vi "ADXL345.vi"() -> ()   [LabVIEW 2012]
uses:
  <vilib>/LabVIEW Interface for Arduino/Type Defs/Board Type.ctl
  <vilib>/LabVIEW Interface for Arduino/LabVIEW Interface for Arduino.lvlib
panel:
  out "Scaled Accelerometer Data":dynamicdata(graph)
  out "Z-Tilt":dbl
  out "Y-Tilt":dbl
  out "X-Tilt":dbl
  out "Raw Accelerometer Data":T1
  in  "Z- Axis Gain":dbl
  in  "Y-Axis Gain":dbl
  in  "X-Axis Gain":dbl
  in  "Board Type (Uno)":T2=enum."Mega 2560"
  in  "Baud Rate (115200)":u32=57600
  in  "COM Port":refnum<visa-resource-name>
  in  "stop":bool
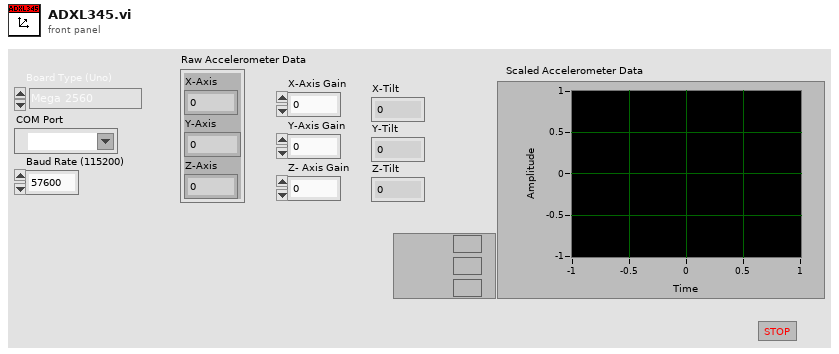
[diagram p1: front panel]
types:
  T1 = cluster{"X-Axis":i32, "Y-Axis":i32, "Z-Axis":i32}
  T2 = typedef "LabVIEW Interface for Arduino.lvlib/Board Type.ctl" = enum16{"Uno", "Dimuelanove w/Atmega 328", "Mega 2560"}
  T3 = typedef "LabVIEW Interface for Arduino.lvlib/Arduino Resource.ctl" = cluster{"VISA resource":refnum<visa-resource-name>, "Board Type":T2, "Connection Type":enum8{"USB / Serial"}, "Bytes Per Packet (15)":u8}
  T4 = cluster{"X-Tilt":dbl, "Y-Tilt":dbl, "Z-Tilt":dbl}
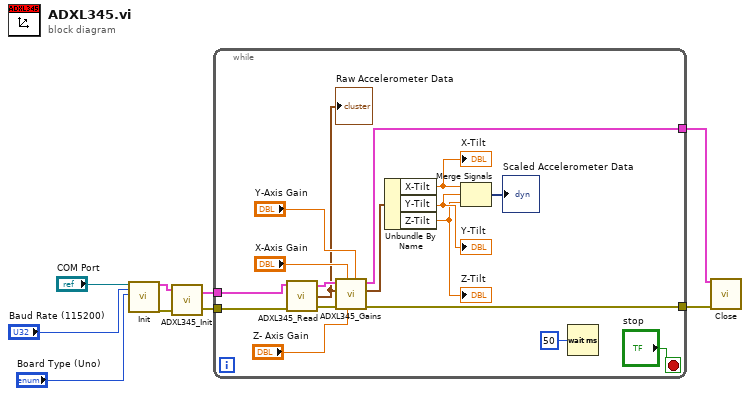
[diagram p0: block diagram]
diagram:
  n1 = call <vilib>:"Init.vi"("VISA resource"="COM Port", "Baud Rate (115200)"="Baud Rate (115200)", "Board Type (Uno)"="Board Type (Uno)") -> ("Arduino Resource"=w6:T3, "error out"=w5:errorcluster)  [unwired: 15 in]
  n2 = call "ADXL345_Init.vi"("error in"=w5, "Arduino Resource"=w6) -> ("error out"=w3:errorcluster, "Arduino Resource"=w4:T3)  [unwired: 1 in]
  n3 = while {
    tunnel: w4 -> [w25]
    tunnel: w3 -> [w24]
    tunnel: [w21] -> w2
    tunnel: [w16] -> w1
    stop <- "stop" stop-if-true
    n4 = call "ADXL345_Read.vi"("error in"=w24, "Arduino Resource"=w25) -> ("error out"=w15:errorcluster, "Raw Accelerometer Data"=w11:T1, "Arduino Resource"=w22:T3)  [unwired: 2 in]
    "Raw Accelerometer Data" <- w11
    n5 = call "ADXL345_Gains.vi"("Y-Axis Gain"="Y-Axis Gain", "Z- Axis Gain"="Z- Axis Gain", "X-Axis Gain"="X-Axis Gain", "error in"=w15, "Raw Accelerometer Data"=w11, "Arduino Resource In"=w22) -> ("error out"=w16:errorcluster, "Tilt Angles"=w20:T4, "Arduino Resource Out"=w21:T3)  [unwired: 3 in]
    n6 = Unbundle By Name(w20) -> ("X-Tilt"=w19:dbl, "Y-Tilt"=w18:dbl, "Z-Tilt"=w17:dbl)
    "X-Tilt" <- w19
    "Y-Tilt" <- w18
    "Z-Tilt" <- w17
    n7 = Merge Signals(w19, w18, w17) -> (→"Scaled Accelerometer Data":dynamicdata)
    n8 = Wait (ms)(milliseconds to wait=u32 50) -> ()  [unwired: 1 out]
  }
  n9 = call <vilib>:"Close.vi"("Arduino Resource"=w2, "error in"=w1) -> ()  [unwired: 13 in, 1 out]
